vi "MT Calculate EbN0.vi"   [LabVIEW 2020, in "niDMT.lvlib"]
doc: "This polymorphic VI estimates the Eb/N0 value of the system from the recieved waveform and the system parameters. The VI performs matched filtering for amplitude modulation based schemes - QAM, PSK, ASK and PAM. Thus, the Eb/N0 estimate is the maximum value seen by the demodulator due to matched filtering."
uses:
  <vilib>/addons/Modulation/niDMT.lvlib
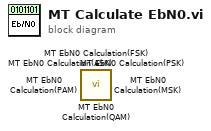
[diagram p0: block diagram]
diagram:
  n1 = call <vilib>:"MT EbN0 Calculation(QAM).vi"() -> ()  [unwired: 13 in, 3 out]
  n2 = call <vilib>:"MT EbN0 Calculation(PSK).vi"() -> ()  [unwired: 13 in, 3 out]
  n3 = call <vilib>:"MT EbN0 Calculation(PAM).vi"() -> ()  [unwired: 13 in, 3 out]
  n4 = call <vilib>:"MT EbN0 Calculation(MSK).vi"() -> ()  [unwired: 13 in, 3 out]
  n5 = call <vilib>:"MT EbN0 Calculation(FSK).vi"() -> ()  [unwired: 13 in, 3 out]
  n6 = call <vilib>:"MT EbN0 Calculation(ASK).vi"() -> ()  [unwired: 13 in, 3 out]
